vi "Load TCP Ports.vi"(8 "error in":errorcluster) -> (0 "error out":errorcluster)   [LabVIEW 2024, in "Data Base.lvlib"]
uses:
  Data Base.lvlib
  <vilib>/Utility/file.llb/Read Delimited Spreadsheet (string).vi
  Support/General Type Defs/Global Data.vi
  Support/General Type Defs/General Type Defs.lvlib
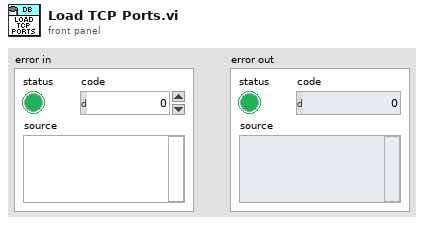
[diagram p1: front panel]
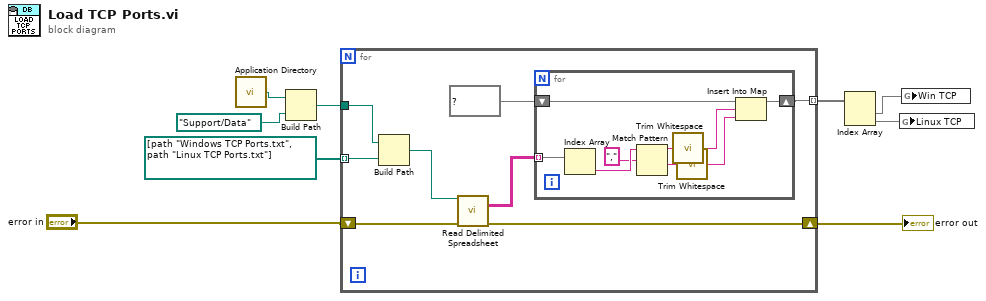
[diagram p0: block diagram]
diagram:
  n1 = call <vilib>:"Application Directory.vi"() -> ("Application Directory"=w9:path)
  n2 = Build Path(base path=w9, name or relative path=path "Support/Data") -> (appended path=w7:path)
  n3 = for {
    tunnel: w7 -> [w17]
    tunnel: path[] [path "Windows TCP Ports.txt", path "Linux TCP Ports.txt"] -> [w14] mode=indexing
    tunnel: [w12] -> w5 mode=indexing
    shift-right: [w11] -> w4
    shift-left: "error in" -> [w10]
    n4 = Build Path(base path=w17, name or relative path=w14) -> (appended path=w16:path)
    n5 = call-poly <vilib>:"Read Delimited Spreadsheet.vi"("file path (dialog if empty)"=w16, "error in (no error)"=w10) -> ("all rows"=w15:string[][], "error out"=w11:errorcluster)  [unwired: 8 in, 4 out]
    n6 = for {
      tunnel: w15 -> [w26] mode=indexing
      shift-right: [w21] -> w12
      shift-left: map{string, string} {} ("map") -> [w23]
      n7 = Index Array(array=w26) -> (element=w25:string)  [unwired: 1 in]
      n8 = Match Pattern(string=w25, regular expression=",") -> (before substring=w22:string, after substring=w20:string)  [unwired: 1 in, 2 out]
      n9 = call <vilib>:"Trim Whitespace.vi"("string"=w22) -> ("trimmed string"=w19:string)  [unwired: 1 in]
      n10 = call <vilib>:"Trim Whitespace.vi"("string"=w20) -> ("trimmed string"=w18:string)  [unwired: 1 in]
      n11 = Insert Into Map(map in=w23, key=w19, value=w18) -> (map out=w21:map{string, string})  [unwired: 2 out]
    }
  }
  "error out" <- w4
  n12 = Index Array(array=w5) -> (element #1=w2:map{string, string}, element #2=w1:map{string, string})  [unwired: 2 in]
  n13 = global write "Global Data.vi" "Linux TCP"(w1) -> ()
  n14 = global write "Global Data.vi" "Win TCP"(w2) -> ()
